vi "Reset.vi"(8 "error in (no error)":errorcluster, 11 "CodeCoverage in":refnum<class "CodeCoverage.lvclass">) -> (0 "error out":errorcluster, 3 "CodeCoverage out":refnum<class "CodeCoverage.lvclass">)   [LabVIEW 2017, in "CodeCoverage.lvclass"]
doc: "Resets code coverage measurements."
uses:
  CodeCoverage.lvclass
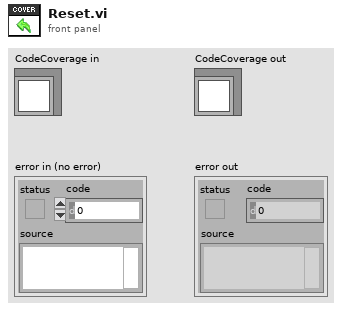
[diagram p1: front panel]
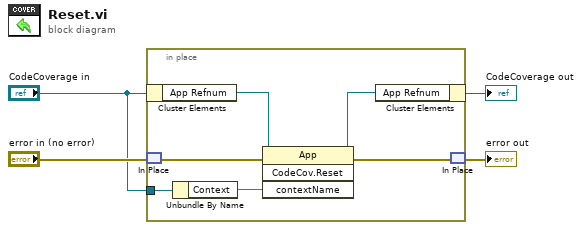
[diagram p0: block diagram]
diagram:
  n1 = in-place {
    in-place-border: "CodeCoverage in" -> [w6]
    n2 = in-place-cluster #1("CodeCoverage in") -> ("App Refnum"=w8:refnum<vi>)
    n3 = in-place-match #2("error in (no error)") -> (w10:errorcluster)
    n4 = Unbundle By Name(w6) -> ("Context"=w5:string)
    n5 = invoke class="App" method="CodeCov.Reset"(reference=w8, error in=w10, "contextName"=w5) -> (reference out=w7:refnum<vi>, error out=w9:errorcluster)  [unwired: 1 in, 2 out]
    n6 = in-place-cluster #1("App Refnum"=w7) -> (→"CodeCoverage out":refnum<class "CodeCoverage.lvclass">)
    n7 = in-place-match #2(w9) -> (→"error out":errorcluster)
  }
